vi "Create Test Configuration.vi"() -> (0 "error out":errorcluster, 1 "Names":string[](array[string]), 2 "Line Array":T1[](array[typedef]) {"Parameters"."Voltage Config"."out terminal configuration (V)" items=["Default"=-1, "RSE"=10083, "Differential"=10106, "Pseudodifferential"=12529]; "Parameters"."Voltage Config"."in terminal configuration (V)" items=["Default"=-1, "RSE"=10083, "NRSE"=10078, "Differential"=10106, "Pseudodifferential"=12529]; "Parameters"."Current Config"."shunt resistor location" items=["default"=-1, "Internal"=10200, "External"=10167]; "Parameters"."Current Config"."input terminal configuration (C)" items=["default"=-1, "RSE"=10083, "NRSE"=10078, "Differential"=10106, "Pseudodifferential"=12529]; "Parameters"."RTD Config"."resistance configuration" items=["2-Wire"=2, "3-Wire"=3, "4-Wire"=4]; "Parameters"."RTD Config"."rtd type" items=["Pt3750"=12481, "Pt3851"=10071, "Pt3911"=12482, "Pt3916"=10069, "Pt3920"=10053, "Pt3928"=12483, "Custom"=10137]; "Parameters"."RTD Config"."current excitation source" items=["Internal"=10200, "External"=10167, "None"=10230]; "Parameters"."Thermocouple Config"."thermocouple type" items=["J"=10072, "K"=10073, "N"=10077, "R"=10082, "S"=10085, "T"=10086, "B"=10047, "E"=10055]; "Parameters"."Thermocouple Config"."cjc source" items=["Built-In"=10200, "Constant Value"=10116, "Channel"=10113]; "Parameters"."Strain Config"."bridge information"."strain configuration" items=["Full Bridge I"=10183, "Full Bridge II"=10184, "Full Bridge III"=10185, "Half Bridge I"=10188, "Half Bridge II"=10189, "Quarter Bridge I"=10271, "Quarter Bridge II"=10272]; "Parameters"."Strain Config"."bridge information"."voltage excitation source" items=["Internal"=10200, "External"=10167, "None"=10230]}, 3 "Module Configuration":refnum<class "Daqmx Module configuration.lvclass">, 4 "Channels":refnum<class "TBM channel.lvclass">[](array[class]), 5 "instance identifier":string)   [LabVIEW 2014, in "DAQmx Module Tests.lvlib"]
doc: "This VI creates a standard test configuration for other unit tests. It currently creates and adds one line with every datatype to the module configuration."
uses:
  DAQmx Module Tests.lvlib
  module/configuration/Daqmx Module configuration.lvclass
  module/configuration/Line.ctl
  <vilib>/NI/Tag Bus Module Framework/channel/TBM channel.lvclass
  module/configuration/Measurement Type.ctl
  module/configuration/Parameters.ctl
  module/configuration/Write Data Rate.vi
  <vilib>/NI/Configuration Framework/serializable configuration/NISE_CEF_serializable configuration.lvclass
  editor node/DAQmx Module editor node.lvclass
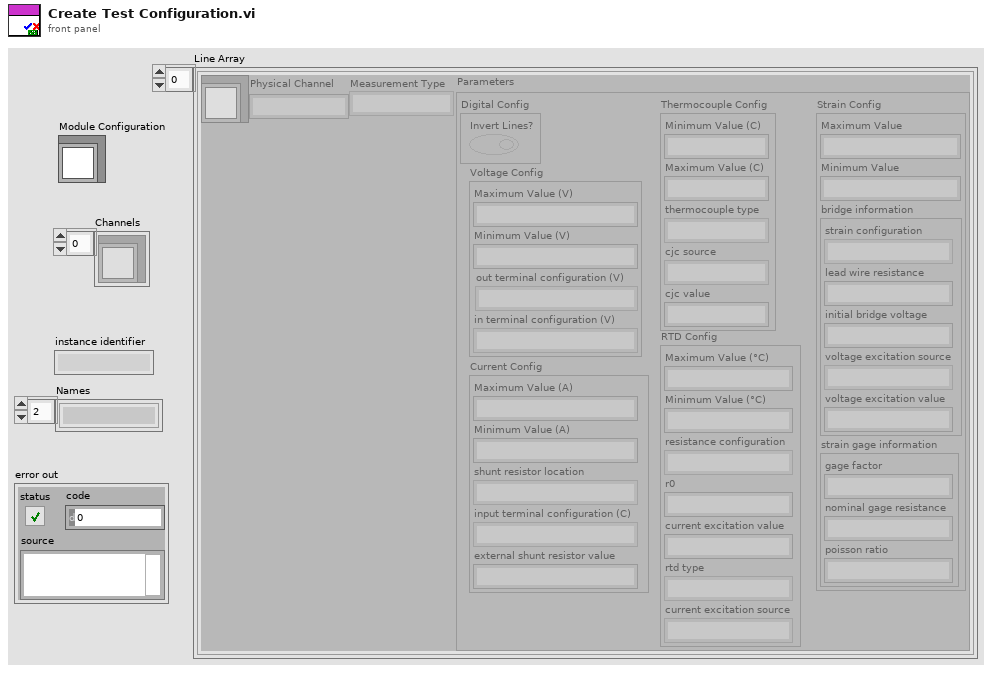
[diagram p1: front panel]
types:
  T1 = typedef "DAQmx Module Configuration.lvclass/Line.ctl" = cluster{"channel":refnum<class "TBM channel.lvclass">, "Physical Channel":string, "Measurement Type":T2, "Parameters":T3}
  T2 = typedef "DAQmx Module Configuration.lvclass/Measurement Type.ctl" = enum16{"Digital Input", "Digital Output", "Voltage Input", "Voltage Output", "Current Input", "Current Output", "RTD", "Thermocouple", "Strain"}
  T3 = typedef "DAQmx Module Configuration.lvclass/Parameters.ctl" = cluster{"Digital Config":cluster{"Invert Lines?":bool}, "Voltage Config":cluster{"Maximum Value (V)":dbl, "Minimum Value (V)":dbl, "in terminal configuration (V)":i32, "out terminal configuration (V)":i32}, "Current Config":cluster{"Maximum Value (A)":dbl, "Minimum Value (A)":dbl, "shunt resistor location":i32, "input terminal configuration (C)":i32, "external shunt resistor value":dbl}, "RTD Config":cluster{"Maximum Value (°C)":dbl, "Minimum Value (°C)":dbl, "resistance configuration":i32, "r0":dbl, "current excitation value":dbl, "rtd type":i32, "current excitation source":i32}, "Thermocouple Config":cluster{"Minimum Value (C)":dbl, "Maximum Value (C)":dbl, "thermocouple type":i32, "cjc source":i32, "cjc value":dbl}, "Strain Config":cluster{"Maximum Value":dbl, "Minimum Value":dbl, "bridge information":cluster{"strain configuration":i32, "lead wire resistance":dbl, "initial bridge voltage":dbl, "voltage excitation source":i32, "voltage excitation value":dbl}, "strain gage information":cluster{"gage factor":dbl, "nominal gage resistance":dbl, "poisson ratio":dbl}}}
  T4 = cluster{"Maximum Value (V)":dbl, "Minimum Value (V)":dbl, "in terminal configuration (V)":i32, "out terminal configuration (V)":i32}
  T5 = cluster{"Maximum Value (A)":dbl, "Minimum Value (A)":dbl, "shunt resistor location":i32, "input terminal configuration (C)":i32, "external shunt resistor value":dbl}
  T6 = cluster{"Maximum Value (°C)":dbl, "Minimum Value (°C)":dbl, "resistance configuration":i32, "r0":dbl, "current excitation value":dbl, "rtd type":i32, "current excitation source":i32}
  T7 = cluster{"Minimum Value (C)":dbl, "Maximum Value (C)":dbl, "thermocouple type":i32, "cjc source":i32, "cjc value":dbl}
  T8 = cluster{"Maximum Value":dbl, "Minimum Value":dbl, "bridge information":cluster{"strain configuration":i32, "lead wire resistance":dbl, "initial bridge voltage":dbl, "voltage excitation source":i32, "voltage excitation value":dbl}, "strain gage information":cluster{"gage factor":dbl, "nominal gage resistance":dbl, "poisson ratio":dbl}}
  T9 = typedef "TBM channel.lvclass/channel classification.ctl" = enum16{"input data", "output data", "processing parameter", "processing result"}
  T10 = typedef "tag bus.lvlib/tag descriptor.lvclass/Data Type.ctl" = enum16{"Double", "Single", "I64", "I32", "I16", "I8", "U64", "U32", "U16", "U8", "Boolean", "String", "Array of Double", "Array of Single", "Array of I64", "Array of I32", "Array of I16", "Array of I8", "Array of U64", "Array of U32", "Array of U16", "Array of U8", "Array of Boolean", "Array of String"}
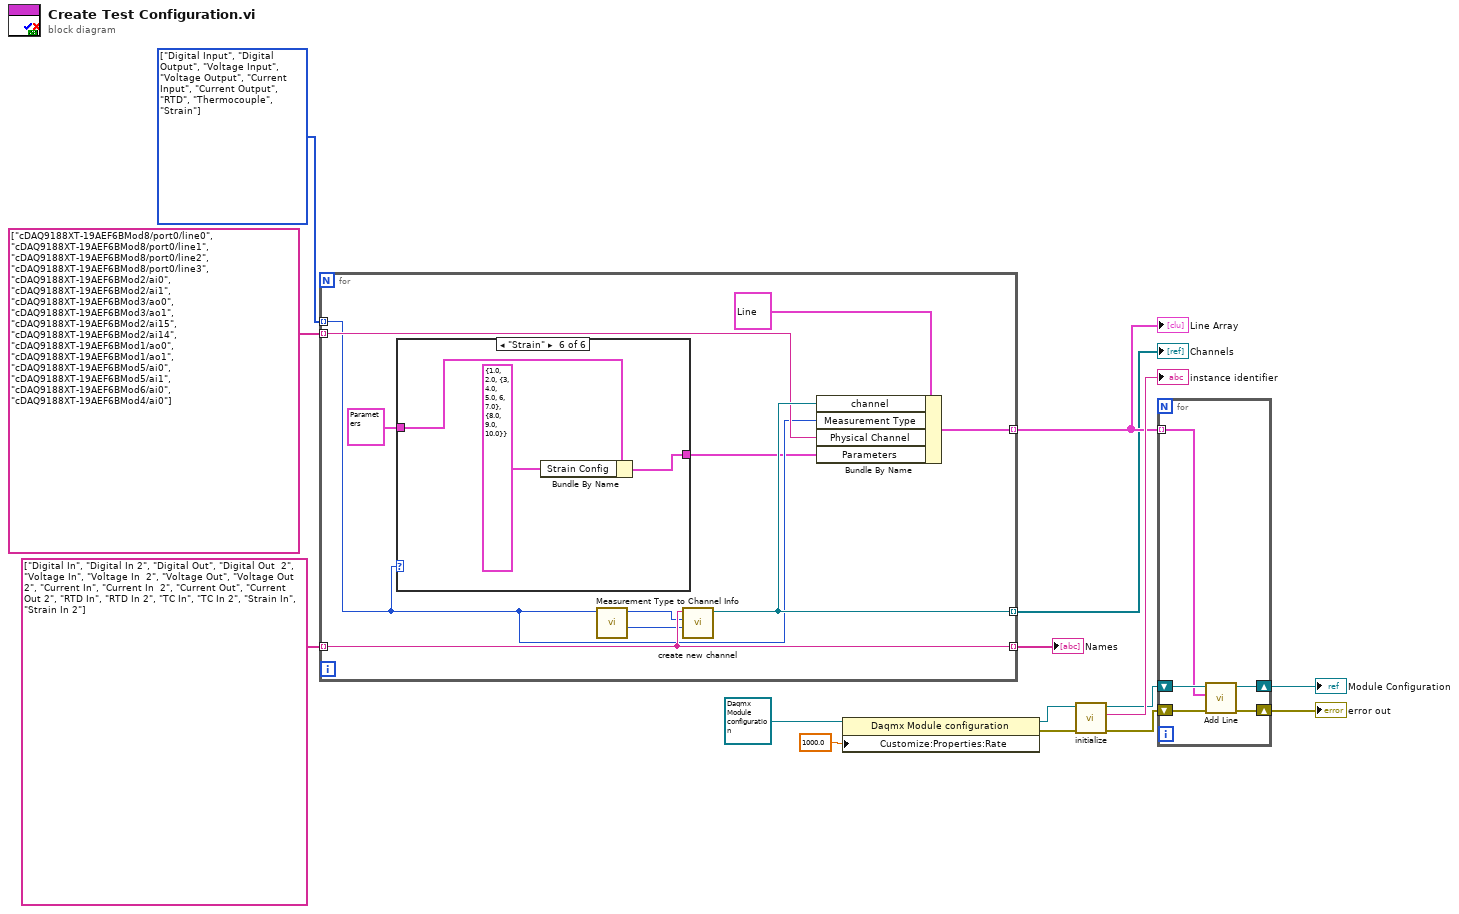
[diagram p0: block diagram]
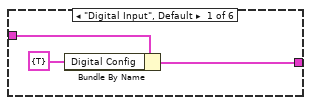
[diagram p2: hidden frame]
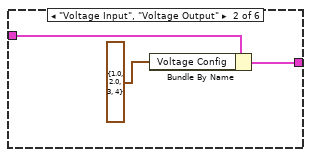
[diagram p3: hidden frame]
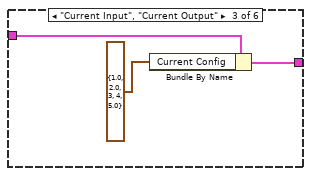
[diagram p4: hidden frame]
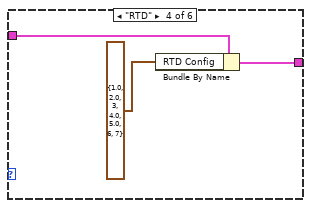
[diagram p5: hidden frame]
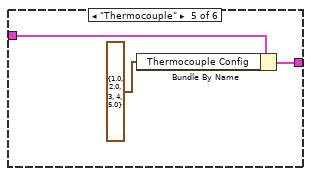
[diagram p6: hidden frame]
diagram:
  w5 = T2[] [enum."Digital Input", enum."Digital Output", enum."Voltage Input", enum."Voltage Output", enum."Current Input", enum."Current Output", enum."RTD", enum."Thermocouple", enum."Strain"] items=["Digital Input", "Digital Output", "Voltage Input", "Voltage Output", "Current Input", "Current Output", "RTD", "Thermocouple", "Strain"]
  n1 = for {
    tunnel: [w24] -> w11 mode=indexing
    tunnel: [w22] -> w12 mode=indexing
    tunnel: [w23] -> w8 mode=indexing
    tunnel: string[] ["Digital In", "Digital In 2", "Digital Out", "Digital Out  2", "Voltage In", "Voltage In  2", "Voltage Out", "Voltage Out  2", "Current In", "Current In  2", "Current Out", "Current Out 2", "RTD In", "RTD In 2", "TC In", "TC In 2", "Strain In", "Strain In 2"] -> [w22] mode=indexing
    tunnel: tag[] ["cDAQ9188XT-19AEF6BMod8/port0/line0", "cDAQ9188XT-19AEF6BMod8/port0/line1", "cDAQ9188XT-19AEF6BMod8/port0/line2", "cDAQ9188XT-19AEF6BMod8/port0/line3", "cDAQ9188XT-19AEF6BMod2/ai0", "cDAQ9188XT-19AEF6BMod2/ai1", "cDAQ9188XT-19AEF6BMod3/ao0", "cDAQ9188XT-19AEF6BMod3/ao1", "cDAQ9188XT-19AEF6BMod2/ai15", "cDAQ9188XT-19AEF6BMod2/ai14", "cDAQ9188XT-19AEF6BMod1/ao0", "cDAQ9188XT-19AEF6BMod1/ao1", "cDAQ9188XT-19AEF6BMod5/ai0", "cDAQ9188XT-19AEF6BMod5/ai1", "cDAQ9188XT-19AEF6BMod6/ai0", "cDAQ9188XT-19AEF6BMod4/ai0"] -> [w21] mode=indexing
    tunnel: w5 -> [w18] mode=indexing
    n2 = case shown="\"Strain\"" w18 {
      tunnel: T3 {"Digital Config"={"Invert Lines?"=FALSE}, "Voltage Config"={"Maximum Value (V)"=5.0, "Minimum Value (V)"=-5.0, "in terminal configuration (V)"=-1, "out terminal configuration (V)"=-1}, "Current Config"={"Maximum Value (A)"=0.02, "Minimum Value (A)"=0.0, "shunt resistor location"=-1, "input terminal configuration (C)"=-1, "external shunt resistor value"=249.0}, "RTD Config"={"Maximum Value (°C)"=100.0, "Minimum Value (°C)"=0.0, "resistance configuration"=2, "r0"=100.0, "current excitation value"=0.0025, "rtd type"=10137, "current excitation source"=10167}, "Thermocouple Config"={"Minimum Value (C)"=0.0, "Maximum Value (C)"=100.0, "thermocouple type"=10072, "cjc source"=10116, "cjc value"=25.0}, "Strain Config"={"Maximum Value"=0.001, "Minimum Value"=-0.001, "bridge information"={"strain configuration"=10183, "lead wire resistance"=0.0, "initial bridge voltage"=0.0, "voltage excitation source"=10200, "voltage excitation value"=2.5}, "strain gage information"={"gage factor"=2.0, "nominal gage resistance"=350.0, "poisson ratio"=0.3}}} ("Parameters") -> [w28 w31 w34 w37 w40 w43]
      tunnel: [w27 w30 w33 w36 w39 w42] -> w16
      frame "Digital Input", Default {
        n3 = Bundle By Name(cluster=w28, "Digital Config"=cluster{"Invert Lines?":bool} {"Invert Lines?"=TRUE}) -> (w27:T3)
      }
      frame "Voltage Input", "Voltage Output" {
        n4 = Bundle By Name(cluster=w31, "Voltage Config"=T4 {"Maximum Value (V)"=1.0, "Minimum Value (V)"=2.0, "in terminal configuration (V)"=3, "out terminal configuration (V)"=4}) -> (w30:T3)
      }
      frame "Current Input", "Current Output" {
        n5 = Bundle By Name(cluster=w34, "Current Config"=T5 {"Maximum Value (A)"=1.0, "Minimum Value (A)"=2.0, "shunt resistor location"=3, "input terminal configuration (C)"=4, "external shunt resistor value"=5.0}) -> (w33:T3)
      }
      frame "RTD" {
        n6 = Bundle By Name(cluster=w37, "RTD Config"=T6 {"Maximum Value (°C)"=1.0, "Minimum Value (°C)"=2.0, "resistance configuration"=3, "r0"=4.0, "current excitation value"=5.0, "rtd type"=6, "current excitation source"=7}) -> (w36:T3)
      }
      frame "Thermocouple" {
        n7 = Bundle By Name(cluster=w40, "Thermocouple Config"=T7 {"Minimum Value (C)"=1.0, "Maximum Value (C)"=2.0, "thermocouple type"=3, "cjc source"=4, "cjc value"=5.0}) -> (w39:T3)
      }
      frame "Strain" {
        n8 = Bundle By Name(cluster=w43, "Strain Config"=T8 {"Maximum Value"=1.0, "Minimum Value"=2.0, "bridge information"={"strain configuration"=3, "lead wire resistance"=4.0, "initial bridge voltage"=5.0, "voltage excitation source"=6, "voltage excitation value"=7.0}, "strain gage information"={"gage factor"=8.0, "nominal gage resistance"=9.0, "poisson ratio"=10.0}}) -> (w42:T3)
      }
    }
    n9 = call "Measurement Type to Channel Info.vi"("Measurement Type"=w18) -> ("channel classification"=w20:T9, "Data Type"=w19:T10)  [unwired: 8 in]
    n10 = call <vilib>:"create new channel.vi"("channel classification"=w20, "data type"=w19, "channel name"=w22) -> ("channel"=w23:refnum<class "TBM channel.lvclass">)  [unwired: 8 in]
    n11 = Bundle By Name(cluster=T1 {"channel"=refnum, "Physical Channel"="", "Measurement Type"=enum."Digital Input", "Parameters"={"Digital Config"={"Invert Lines?"=FALSE}, "Voltage Config"={"Maximum Value (V)"=5.0, "Minimum Value (V)"=-5.0, "in terminal configuration (V)"=-1, "out terminal configuration (V)"=-1}, "Current Config"={"Maximum Value (A)"=0.02, "Minimum Value (A)"=0.0, "shunt resistor location"=-1, "input terminal configuration (C)"=-1, "external shunt resistor value"=249.0}, "RTD Config"={"Maximum Value (°C)"=100.0, "Minimum Value (°C)"=0.0, "resistance configuration"=2, "r0"=100.0, "current excitation value"=0.0025, "rtd type"=10137, "current excitation source"=10167}, "Thermocouple Config"={"Minimum Value (C)"=0.0, "Maximum Value (C)"=100.0, "thermocouple type"=10072, "cjc source"=10116, "cjc value"=25.0}, "Strain Config"={"Maximum Value"=0.001, "Minimum Value"=-0.001, "bridge information"={"strain configuration"=10183, "lead wire resistance"=0.0, "initial bridge voltage"=0.0, "voltage excitation source"=10200, "voltage excitation value"=2.5}, "strain gage information"={"gage factor"=2.0, "nominal gage resistance"=350.0, "poisson ratio"=0.3}}}} ("Line"), "channel"=w23, "Measurement Type"=w18, "Physical Channel"=w21, "Parameters"=w16) -> (w24:T1)
  }
  "Names" <- w12
  "Line Array" <- w11
  "Channels" <- w8
  n12 = property class="Daqmx Module configuration"(reference=refnum<class "Daqmx Module configuration.lvclass"> refnum ("tag bus configurable plugin module configuration"), "Customize:Properties:Rate"=1000.0 ("Rate")) -> (reference out=w3:refnum<class "Daqmx Module configuration.lvclass">, error out=w2:errorcluster)  [unwired: 1 in]
  n13 = call <vilib>:"initialize.vi"("error in"=w2, "configuration in"=w3) -> ("error out"=w13:errorcluster, "identifier"=→"instance identifier":string, "configuration out"=w9:refnum<class "Daqmx Module configuration.lvclass">)  [unwired: 7 in]
  n14 = for {
    tunnel: w11 -> [w44] mode=indexing
    shift-right: [w47] -> w10
    shift-left: w9 -> [w48]
    shift-right: [w45] -> w15
    shift-left: w13 -> [w46]
    n15 = call "Add Line.vi"("error in"=w46, "Line"=w44, "Daqmx Module configuration in"=w48) -> ("error out"=w45:errorcluster, "Daqmx Module configuration out"=w47:refnum<class "Daqmx Module configuration.lvclass">)  [unwired: 6 in, 1 out]
  }
  "error out" <- w15
  "Module Configuration" <- w10
